vi "Multiple_Thread_Client.vi"() -> ()   [LabVIEW 2021]
panel:
  out "Active 1":bool=TRUE
  out "Active 0":bool=TRUE
  in  "error in (no error) 2":errorcluster
  in  "Stop 1":bool
  in  "Send 1":bool
  out "Data out 1":string
  out "error out 2":errorcluster
  out "error out":errorcluster
  in  "Stop 0":bool
  in  "Send 0":bool
  out "Data out 0":string
  in  "error in (no error)":errorcluster
  # "Socket 0"
  # "Socket 1"
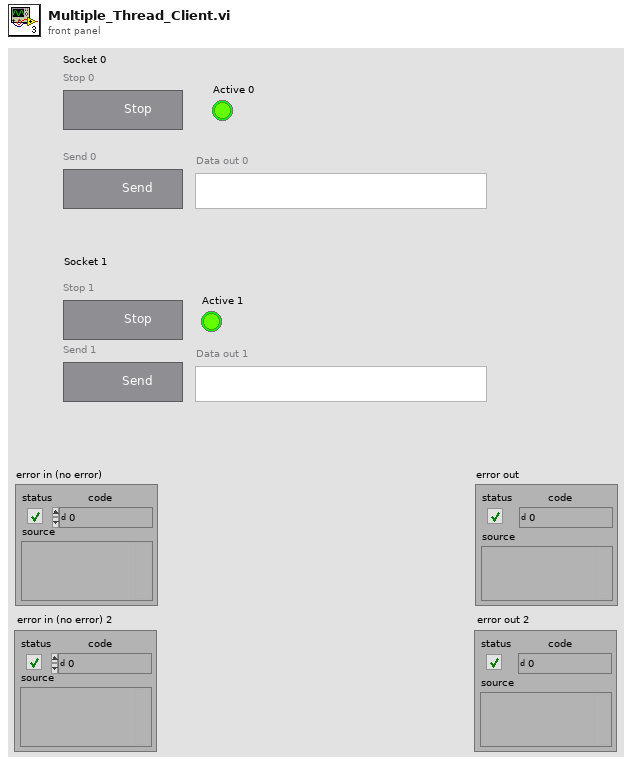
[diagram p1: front panel]
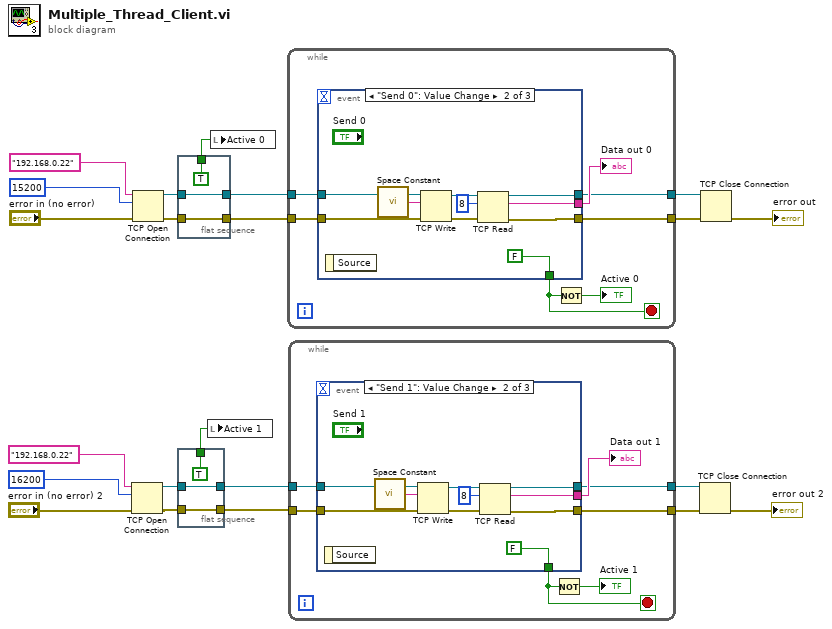
[diagram p0: block diagram]
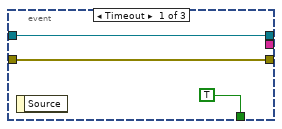
[diagram p2: hidden frame]
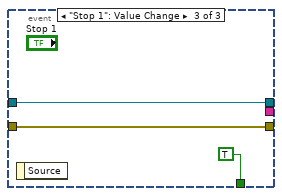
[diagram p3: hidden frame]
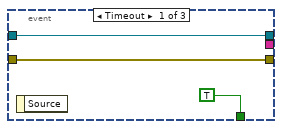
[diagram p4: hidden frame]
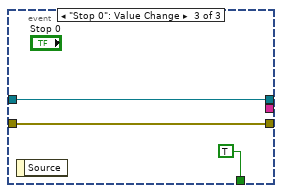
[diagram p5: hidden frame]
diagram:
  n1 = TCP Open Connection(address="192.168.0.22", remote port or service name=u16 16200, error in (no error)="error in (no error) 2") -> (connection ID=w2:refnum<k5>, error out=w4:errorcluster)  [unwired: 2 in]
  n2 = TCP Open Connection(address="192.168.0.22", remote port or service name=u16 15200, error in (no error)="error in (no error)") -> (connection ID=w9:refnum<k5>, error out=w7:errorcluster)  [unwired: 2 in]
  n3 = flat-sequence {
    tunnel: [w25] -> w10
    tunnel: w9 -> [w25]
    tunnel: [w24] -> w8
    tunnel: w7 -> [w24]
    tunnel: [TRUE] -> w6
    frame #0 {
    }
  }
  n4 = flat-sequence {
    tunnel: [w28] -> w5
    tunnel: w4 -> [w28]
    tunnel: [w27] -> w3
    tunnel: w2 -> [w27]
    tunnel: [TRUE] -> w1
    frame #0 {
    }
  }
  n5 = local write "Active 1"(w1) -> ()
  n6 = local write "Active 0"(w6) -> ()
  n7 = while {
    tunnel: w10 -> [w31]
    tunnel: w8 -> [w30]
    tunnel: [w34] -> w19
    tunnel: [w33] -> w17
    stop <- w32 stop-if-true
    n8 = event shown="[1] \"Send 0\": Value Change" {
      selector: _ -> [_ _ _]
      dyn-events: _ -> [_ _ _]
      timeout: _ -> [_ _ _]
      tunnel: w30 -> [w38 w48 w51]
      tunnel: w31 -> [w36 w47 w49]
      tunnel: [_ w44 _] -> w35
      tunnel: [w38 w43 w51] -> w34
      tunnel: [TRUE FALSE TRUE] -> w32
      tunnel: [w36 w41 w49] -> w33
      event Timeout {
        n9 = event-data() -> ()  [unwired: 1 in, 1 out]
      }
      event "Send 0": Value Change {
        n10 = event-data() -> ()  [unwired: 1 in, 1 out]
        n11 = call <vilib>:"Space Constant.vi"() -> ("String"=w39:string)
        n12 = TCP Write(connection ID=w47, data in=w39, error in (no error)=w48) -> (connection ID out=w45:refnum<k5>, error out=w46:errorcluster)  [unwired: 1 in, 1 out]
        n13 = TCP Read(connection ID=w45, bytes to read=8, error in (no error)=w46) -> (connection ID out=w41:refnum<k5>, data out=w44:string, error out=w43:errorcluster)  [unwired: 2 in]
      }
      event "Stop 0": Value Change {
        n14 = event-data() -> ()  [unwired: 1 in, 1 out]
      }
    }
    "Data out 0" <- w35
    n15 = Not(x=w32) -> (.not. x?=→"Active 0":bool)
  }
  n16 = while {
    tunnel: w3 -> [w57]
    tunnel: w5 -> [w58]
    tunnel: [w55] -> w14
    tunnel: [w54] -> w16
    stop <- w53 stop-if-true
    n17 = event shown="[1] \"Send 1\": Value Change" {
      selector: _ -> [_ _ _]
      dyn-events: _ -> [_ _ _]
      timeout: _ -> [_ _ _]
      tunnel: w58 -> [w61 w71 w74]
      tunnel: w57 -> [w59 w70 w72]
      tunnel: [_ w67 _] -> w56
      tunnel: [w61 w66 w74] -> w55
      tunnel: [TRUE FALSE TRUE] -> w53
      tunnel: [w59 w64 w72] -> w54
      event Timeout {
        n18 = event-data() -> ()  [unwired: 1 in, 1 out]
      }
      event "Send 1": Value Change {
        n19 = event-data() -> ()  [unwired: 1 in, 1 out]
        n20 = call <vilib>:"Space Constant.vi"() -> ("String"=w62:string)
        n21 = TCP Write(connection ID=w70, data in=w62, error in (no error)=w71) -> (connection ID out=w68:refnum<k5>, error out=w69:errorcluster)  [unwired: 1 in, 1 out]
        n22 = TCP Read(connection ID=w68, bytes to read=8, error in (no error)=w69) -> (connection ID out=w64:refnum<k5>, data out=w67:string, error out=w66:errorcluster)  [unwired: 2 in]
      }
      event "Stop 1": Value Change {
        n23 = event-data() -> ()  [unwired: 1 in, 1 out]
      }
    }
    "Data out 1" <- w56
    n24 = Not(x=w53) -> (.not. x?=→"Active 1":bool)
  }
  n25 = TCP Close Connection(connection ID=w16, error in (no error)=w14) -> (error out=→"error out 2":errorcluster)  [unwired: 1 in, 1 out]
  n26 = TCP Close Connection(connection ID=w17, error in (no error)=w19) -> (error out=→"error out":errorcluster)  [unwired: 1 in, 1 out]
